vi "Go_to_Saved_Position.vi"(6 "Echo Mode":i32, 7 "file path (use dialog)":path, 8 "error in":errorcluster={"status"=FALSE, "code"=1073676294, "source"="VISA Read in write_read.vi"}, 11 "ComPort":refnum<visa-resource-name>="COM11") -> (0 "error out":errorcluster={"status"=FALSE, "code"=1073676294, "source"="VISA Read in write_read.vi"}, 2 "Loaded Positions":string, 3 "VISA ressource out":refnum<visa-resource-name>)   [LabVIEW 2018]
uses:
  MCode_LV_86/Set Parameter.ctl
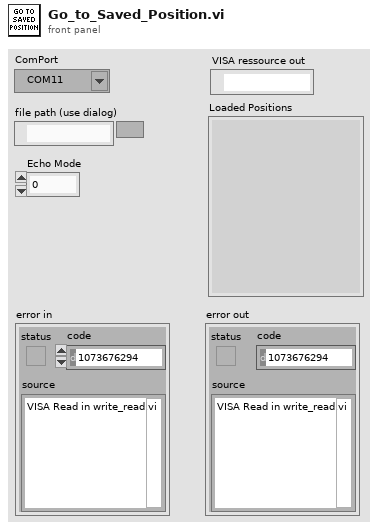
[diagram p1: front panel]
types:
  T1 = typedef "Set Parameter.ctl" = enum16{"Acceleration (A)", "Baud Rate (BD)", "Counter 1 (C1)", "Counter 2 (C2)", "Control C Software Reset (CE)", "Check Sum Enable (CK)", "Clock Mode (CM)", "Clock Mode Ratio (CR)", "Clock Mode Out Step Width (CW)", "Deceleration (D)", "Digital Filtering, Input 1 (D1)", "Digital Filtering, Input 2 (D2)", "Digital Filtering, Input 3 (D3)", "Digital Filtering, Input 4 (D4)", "Digital Filtering, Input 5 (D5)", "Digital Filtering, Input 9 (D9)", "Digital Filtering, Input 10 (D10)", "Digital Filtering, Input 11 (D11)", "Digital Filtering, Input 12 (D12)", "Deadband (DB)", "Decrement Variable (DC)", "Enable/Disable Drive (DE)", "Device Name (DN)", "End Program Execution (E)", "Encoder Function Enable (EE)", "Error Flag (EF)", "Encoder Lines (EL)", "Echo Mode (EM)", "Error Value (ER)", "Escape (ES)", "Execute Program at Address (EX)", "Firmware Version (VR)", "Hold (H)", "Hold Current (HC)", "Hold Current Delay Time (HI)", "Home to Encoder Index (HM)", "Home to Home Switch (HT)", "Increment Variable (IC)", "Initialize Parameters to NVM (IP)", "Input into Variable (IV)", "Jog Enable (JE)", "Limit Stop Mode (LM)", "Move Absolute (MA)", "Move Relative (MR)", "MicroStepping Select (MS)", "Motor Settling Delay Time (MT)", "Moving [Flag] (MV)", "Output 1 (O1)", "Output 2 (O2)", "Output 3 (O3)", "Output 4 (O4)", "Output 9 (O9)", "Output 10 (O10)", "Output 11 (O11)", "Output 12 (O12)", "Output High Byte (9-12) (OH)", "Output Low Byte (1-4) (OL)", "Output Total (1-4 and 9-12) (OT)", "Position (P)", "Position Maintenance (PM)", "Party Mode (PY)", "Register 1 (R1)", "Register 2 (R2)", "Register 3 (R3)", "Register 4 (R4)", "Reset Error(\\03)", "Run Current (RC)", "Stall Factor (SF)", "Slew (SL)", "Stall Mode Set (SM)", "Upgrade Firmware (UG)", "Velocity Initial (VI)", "Velocity Maximum (VM)", "Current1 (I1)", "Current2 (I2)", "Current3 (I3)", "Current4 (I4)", "Current5 (I5)", "Current6 (I6)", "Save (S)"}
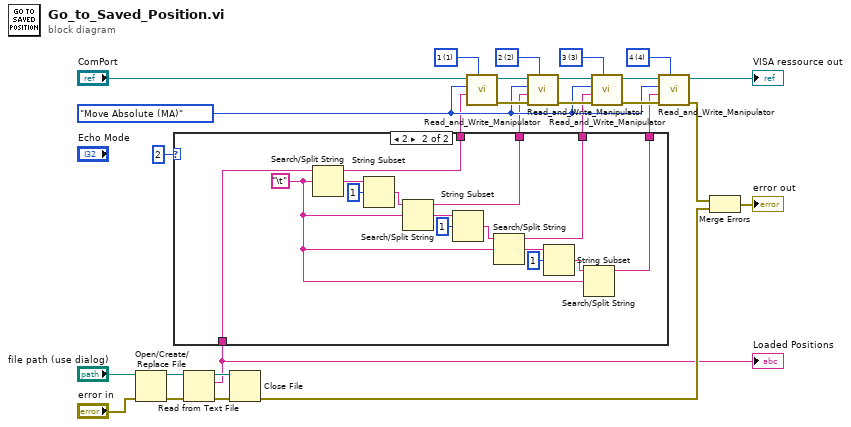
[diagram p0: block diagram]
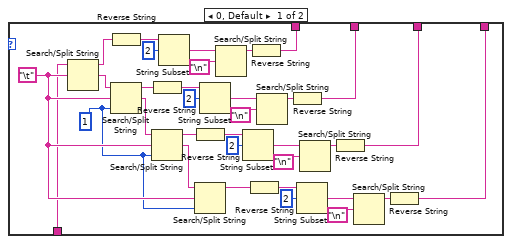
[diagram p2: hidden frame]
diagram:
  w18 = u16 4 items=["none", "1", "2", "3", "4", "all"] ("Motor")
  w19 = u16 3 items=["none", "1", "2", "3", "4", "all"] ("Motor")
  w20 = u16 2 items=["none", "1", "2", "3", "4", "all"] ("Motor")
  w21 = u16 1 items=["none", "1", "2", "3", "4", "all"] ("Motor")
  w22 = Set_Parameter."Move Absolute (MA)" ("Command")
  n1 = Open/Create/Replace File(file path (use dialog)="file path (use dialog)", error in="error in") -> (refnum out=w15:refnum<file>, error out=w14:errorcluster)  [unwired: 4 in, 1 out]
  n2 = Read from Text File(file (use dialog)=w15, error in=w14) -> (refnum out=w13:refnum<file>, text=w2:string, error out=w12:errorcluster)  [unwired: 2 in, 1 out]
  "Loaded Positions" <- w2
  n3 = case shown="2" 2 ("Echo Mode") {
    tunnel: [w33 w76] -> w9
    tunnel: [w32 w75] -> w8
    tunnel: [w31 w74] -> w7
    tunnel: [w30 w73] -> w6
    tunnel: w2 -> [w29 w77]
    frame 0, Default {
      w58 = 1 ("offset (0)")
      w59 = "\t"
      n4 = Search/Split String(string=w29, search string/char (-)=w59) -> (substring before match=w57:string, match + rest of string=w62:string)  [unwired: 1 in, 1 out]
      n5 = Reverse String(1:w57) -> (0:w56:string)
      n6 = Search/Split String(string=w62, search string/char (-)=w59, offset (0)=w58) -> (substring before match=w36:string, match + rest of string=w61:string)  [unwired: 1 out]
      n7 = Reverse String(1:w36) -> (0:w47:string)
      n8 = Search/Split String(string=w61, search string/char (-)=w59, offset (0)=w58) -> (substring before match=w35:string, match + rest of string=w60:string)  [unwired: 1 out]
      n9 = String Subset(string=w56, offset (0)=2) -> (substring=w53:string)  [unwired: 1 in]
      n10 = Reverse String(1:w35) -> (0:w46:string)
      n11 = Search/Split String(string=w60, search string/char (-)=w59, offset (0)=w58) -> (substring before match=w34:string)  [unwired: 2 out]
      n12 = String Subset(string=w47, offset (0)=2) -> (substring=w50:string)  [unwired: 1 in]
      n13 = Search/Split String(string=w53, search string/char (-)="\n") -> (substring before match=w52:string)  [unwired: 1 in, 2 out]
      n14 = String Subset(string=w46, offset (0)=2) -> (substring=w43:string)  [unwired: 1 in]
      n15 = Reverse String(1:w34) -> (0:w37:string)
      n16 = Reverse String(1:w52) -> (0:w33:string)
      n17 = Search/Split String(string=w50, search string/char (-)="\n") -> (substring before match=w51:string)  [unwired: 1 in, 2 out]
      n18 = Reverse String(1:w51) -> (0:w32:string)
      n19 = String Subset(string=w37, offset (0)=2) -> (substring=w40:string)  [unwired: 1 in]
      n20 = Search/Split String(string=w43, search string/char (-)="\n") -> (substring before match=w42:string)  [unwired: 1 in, 2 out]
      n21 = Reverse String(1:w42) -> (0:w31:string)
      n22 = Search/Split String(string=w40, search string/char (-)="\n") -> (substring before match=w41:string)  [unwired: 1 in, 2 out]
      n23 = Reverse String(1:w41) -> (0:w30:string)
    }
    frame 2 {
      w63 = "\t"
      n24 = Search/Split String(string=w77, search string/char (-)=w63) -> (substring before match=w76:string, match + rest of string=w72:string)  [unwired: 1 in, 1 out]
      n25 = String Subset(string=w72, offset (0)=1) -> (substring=w71:string)  [unwired: 1 in]
      n26 = Search/Split String(string=w71, search string/char (-)=w63) -> (substring before match=w75:string, match + rest of string=w69:string)  [unwired: 1 in, 1 out]
      n27 = String Subset(string=w69, offset (0)=1) -> (substring=w68:string)  [unwired: 1 in]
      n28 = Search/Split String(string=w68, search string/char (-)=w63) -> (substring before match=w74:string, match + rest of string=w65:string)  [unwired: 1 in, 1 out]
      n29 = String Subset(string=w65, offset (0)=1) -> (substring=w64:string)  [unwired: 1 in]
      n30 = Search/Split String(string=w64, search string/char (-)=w63) -> (substring before match=w73:string)  [unwired: 1 in, 2 out]
    }
  }
  n31 = Close File(refnum=w13, error in=w12) -> (error out=w4:errorcluster)  [unwired: 1 out]
  n32 = call "Read_and_Write_Manipulator.vi"("Motor"=w21, "Value"=w9, "Command"=w22, "VISA resource name"="ComPort") -> ("error out"=w28:errorcluster, "VISA ressource out"=w25:refnum<visa-resource-name>)  [unwired: 3 in, 3 out]
  n33 = call "Read_and_Write_Manipulator.vi"("Motor"=w20, "error in (no error)"=w28, "Value"=w8, "Command"=w22, "VISA resource name"=w25) -> ("error out"=w27:errorcluster, "VISA ressource out"=w24:refnum<visa-resource-name>)  [unwired: 2 in, 3 out]
  n34 = call "Read_and_Write_Manipulator.vi"("Motor"=w19, "error in (no error)"=w27, "Value"=w7, "Command"=w22, "VISA resource name"=w24) -> ("error out"=w26:errorcluster, "VISA ressource out"=w23:refnum<visa-resource-name>)  [unwired: 2 in, 3 out]
  n35 = call "Read_and_Write_Manipulator.vi"("Motor"=w18, "error in (no error)"=w26, "Value"=w6, "Command"=w22, "VISA resource name"=w23) -> ("error out"=w5:errorcluster, "VISA ressource out"=→"VISA ressource out":refnum<visa-resource-name>)  [unwired: 2 in, 3 out]
  n36 = Merge Errors(w5, w4) -> (→"error out":errorcluster)
